vi "List Status in Registry.vi"(0 "BroadcastRegistry In":T1) -> (4 "BroadcastRegistry Out":T1, 6 "Broadcast":string[](array[string]))   [LabVIEW 2017, in "Communicable State Machine.lvlib"]
doc: "### List Status in Registry.vi\n\n-- <b>Controls</b> --\n- <b>BroadcastRegistry in</b>:\n\n-- <b>Indicators</b> --\n- <b>BroadcastRegistry out</b>:\n- <b>Status</b>:"
uses:
  Communicable State Machine.lvlib
  BroadcastRegistry.ctl
  _Shared/CSM Shared.lvlib
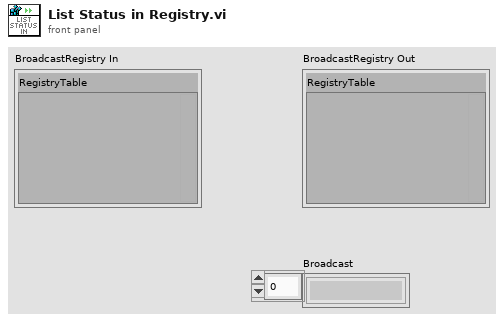
[diagram p1: front panel]
types:
  T1 = typedef "Communicable State Machine.lvlib/BroadcastRegistry.ctl" = cluster{"RegistryTable":variant}
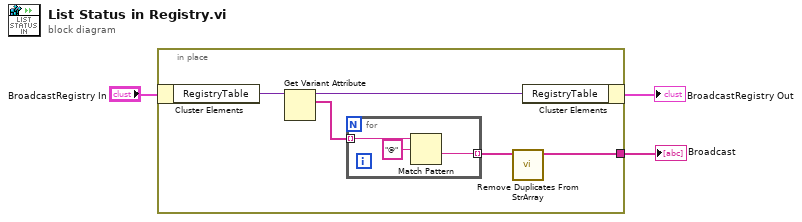
[diagram p0: block diagram]
diagram:
  n1 = in-place {
    in-place-border: [w4] -> w1
    n2 = in-place-cluster #1("BroadcastRegistry In") -> ("RegistryTable"=w8:variant)
    n3 = Get Variant Attribute(Variant=w8) -> (duplicate Variant=w7:variant, names=w6:string[])  [unwired: 3 in, 2 out]
    n4 = for {
      tunnel: w6 -> [w11] mode=indexing
      tunnel: [w9] -> w5 mode=indexing
      n5 = Match Pattern(string=w11, regular expression="@") -> (after substring=w9:string)  [unwired: 1 in, 3 out]
    }
    n6 = call "Remove Duplicates From StrArray.vi"("StrArray In"=w5) -> ("StrArray"=w4:string[])  [unwired: 9 in, 1 out]
    n7 = in-place-cluster #1("RegistryTable"=w7) -> (→"BroadcastRegistry Out":T1)
  }
  "Broadcast" <- w1
